vi "UDPPrototype.vi"() -> ()   [LabVIEW 2013, in "TEC tests.lvlib"]
uses:
  <vilib>/NI/Tag Bus/table/data table.ctl
  <vilib>/NI/Tag Bus/tag/Data Type.ctl
  <vilib>/NI/Tag Bus/tag/tag descriptor.lvclass
  <vilib>/NI/Tag Bus/dictionary/data dictionary.lvclass/data dictionary.ctl
  TEC tests.lvlib
  <vilib>/NI/Tag Bus/dictionary/data dictionary.lvclass
  <vilib>/NI/Tag Bus/table/data table.lvlib
panel:
  out "x = y?":bool
  out "error out":errorcluster
  in  "error in":errorcluster
  in  "Stop 2":bool
  out "Received Data":dbl(graph)
  in  "Stop":bool
  out "Current Data Value":dbl
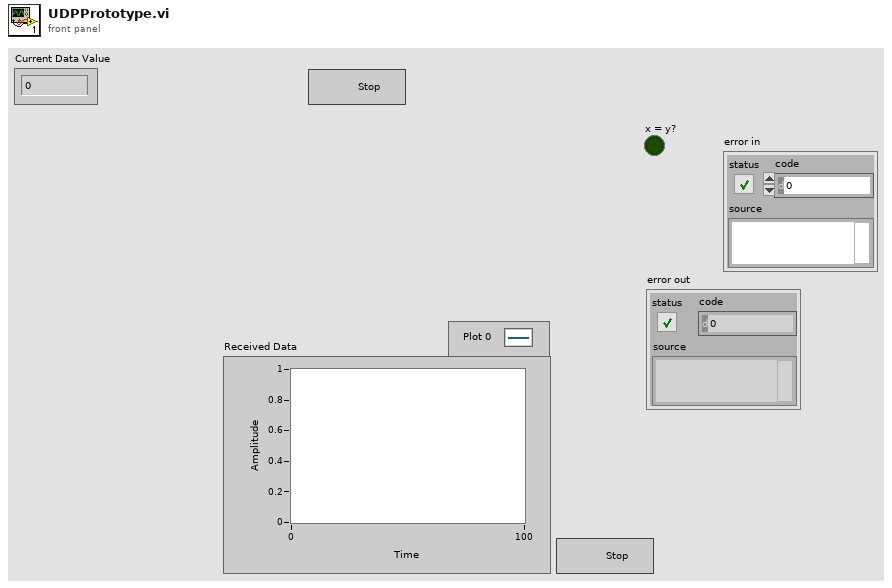
[diagram p1: front panel]
types:
  T1 = typedef "tag bus.lvlib/data table.lvlib/data table.ctl" = cluster{"Double":dbl[], "Single":sgl[], "I64":i64[], "I32":i32[], "I16":i16[], "I8":i8[], "U64":u64[], "U32":u32[], "U16":u16[], "U8":u8[], "Boolean":bool[], "String":string[], "Array of Double":cluster{"DBL Array":dbl[]}[], "Array of Single":cluster{"SGL Array":sgl[]}[], "Array of I64":cluster{"I64 Array":i64[]}[], "Array of I32":cluster{"I32 Array":i32[]}[], "Array of I16":cluster{"I16 Array":i16[]}[], "Array of I8":cluster{"I8 Array":i8[]}[], "Array of U64":cluster{"U64 Array":u64[]}[], "Array of U32":cluster{"U32 Array":u32[]}[], "Array of U16":cluster{"U16 Array":u16[]}[], "Array of U8":cluster{"U8 Array":u8[]}[], "Array of Boolean":cluster{"Boolean Array":bool[]}[], "Array of String":cluster{"String Array":string[]}[]}
  T2 = typedef "tag bus.lvlib/tag descriptor.lvclass/Data Type.ctl" = enum16{"Double", "Single", "I64", "I32", "I16", "I8", "U64", "U32", "U16", "U8", "Boolean", "String", "Array of Double", "Array of Single", "Array of I64", "Array of I32", "Array of I16", "Array of I8", "Array of U64", "Array of U32", "Array of U16", "Array of U8", "Array of Boolean", "Array of String"}
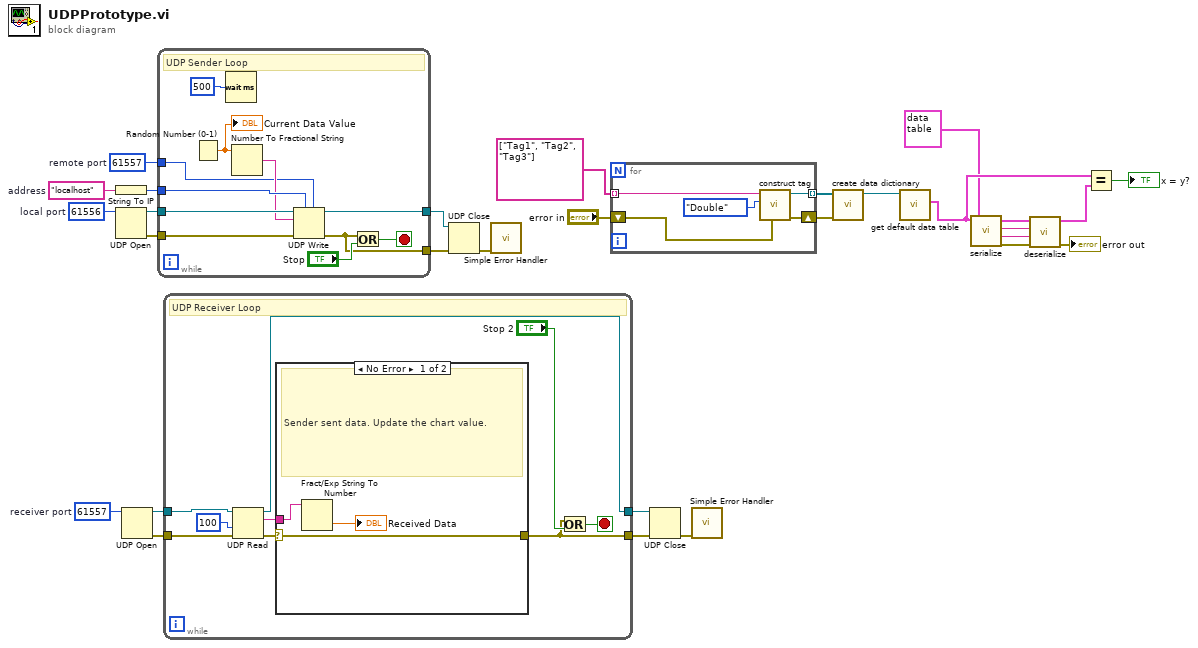
[diagram p0: block diagram]
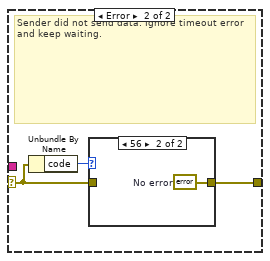
[diagram p2: hidden frame]
diagram:
  w14 = u16 61557  # receiver port
  w20 = u16 61557  # remote port
  w21 = u16 61556  # local port
  w26 = "localhost"  # address
  n1 = String To IP(1:w26) -> (0:w24:u32)
  n2 = UDP Open(11:w21) -> (port=w23:refnum<k16>, 0:w22:errorcluster)  [unwired: 4 in, 1 out]
  n3 = UDP Open(11:w14) -> (port=w15:refnum<k16>, 0:w16:errorcluster)  [unwired: 4 in, 1 out]
  n4 = while {
    tunnel: [w34] -> w27
    tunnel: w23 -> [w39]
    tunnel: w22 -> [w38]
    tunnel: [w35] -> w28
    tunnel: w24 -> [w33]
    tunnel: w20 -> [w30]
    stop <- w37 stop-if-true
    # "UDP Sender Loop"
    n5 = Random Number (0-1)() -> (number: 0 to 1=w29:dbl)
    "Current Data Value" <- w29
    n6 = Wait (ms)(milliseconds to wait=u32 500) -> ()  [unwired: 1 out]
    n7 = Number To Fractional String(number=w29) -> (F-format string=w31:string)  [unwired: 3 in]
    n8 = UDP Write(address=w33, port or service name=w30, connection ID=w39, data in=w31, 8:w38) -> (error out=w34:errorcluster, 3:w35:refnum<k16>)  [unwired: 1 in]
    n9 = Or(x=w34, y="Stop") -> (x .or. y?=w37:bool)
  }
  n10 = while {
    tunnel: w15 -> [w48]
    tunnel: [w40] -> w19
    tunnel: w16 -> [w45]
    tunnel: [w41] -> w17
    stop <- w46 stop-if-true
    # "UDP Receiver Loop"
    n11 = UDP Read(connection ID=w48, timeout ms (25000)=100, 8:w45) -> (data out=w43:string, error out=w42:errorcluster, 3:w40:refnum<k16>)  [unwired: 3 out]
    n12 = case shown="No Error" w42 {
      selector: w42 -> [w49 w53]
      tunnel: w43 -> [w51 _]
      tunnel: [w49 w52] -> w41
      frame No Error {
        # "Sender sent data. Update the chart value."
        n13 = Fract/Exp String To Number(string=w51) -> (number=→"Received Data":dbl)  [unwired: 3 in, 1 out]
      }
      frame Error {
        # "Sender did not send data. Ignore timeout error and keep waiting."
        n14 = Unbundle By Name(w53) -> ("code"=w54:i32)
        n15 = case shown="56" w54 {
          tunnel: w53 -> [w55 _]
          tunnel: [w55 w56] -> w52
          frame Default {
          }
          frame 56 {
            w56 = errorcluster {"status"=FALSE, "code"=0, "source"=""}  # No error
          }
        }
      }
    }
    n16 = Or(x=w41, y="Stop 2") -> (x .or. y?=w46:bool)
  }
  n17 = UDP Close(connection ID=w28, 8:w27) -> (error out=w25:errorcluster)  [unwired: 1 out]
  n18 = call <vilib>:"Simple Error Handler.vi"("error in (no error)"=w25) -> ()  [unwired: 4 in, 5 out]
  n19 = for {
    tunnel: [w61] -> w12 mode=indexing
    tunnel: string[] ["Tag1", "Tag2", "Tag3"] ("array") -> [w57] mode=indexing
    shift-right: [w58] -> w10
    shift-left: "error in" -> [w59]
    n20 = call <vilib>:"construct tag.vi"("error in"=w59, "data type"=Data_Type."Double", "name"=w57) -> ("error out"=w58:errorcluster, "system tag out"=w61:refnum<class "tag descriptor.lvclass">)  [unwired: 7 in]
  }
  n21 = UDP Close(connection ID=w19, 8:w17) -> (error out=w18:errorcluster)  [unwired: 1 out]
  n22 = call <vilib>:"Simple Error Handler.vi"("error in (no error)"=w18) -> ()  [unwired: 1 in, 8 out]
  n23 = call <vilib>:"create data dictionary.vi"("error in"=w10, "system tags"=w12) -> ("data dictionary"=w13:refnum<class "data dictionary.lvclass">)  [unwired: 8 in, 1 out]
  n24 = call <vilib>:"get default data table.vi"("data dictionary in"=w13) -> ("default data table"=w3:T1)  [unwired: 9 in, 1 out]
  n25 = call <vilib>:"serialize.vi"("data table in"=w3) -> ("error out"=w8:errorcluster, "data"=w6:string, "version"=w7:string)  [unwired: 7 in, 1 out]
  n26 = call <vilib>:"deserialize.vi"("error in"=w8, "data"=w6, "version"=w7, "data table in"=T1 {"Double"=[], "Single"=[], "I64"=[], "I32"=[], "I16"=[], "I8"=[], "U64"=[], "U32"=[], "U16"=[], "U8"=[], "Boolean"=[], "String"=[], "Array of Double"=[], "Array of Single"=[], "Array of I64"=[], "Array of I32"=[], "Array of I16"=[], "Array of I8"=[], "Array of U64"=[], "Array of U32"=[], "Array of U16"=[], "Array of U8"=[], "Array of Boolean"=[], "Array of String"=[]}) -> ("error out"=→"error out":errorcluster, "data table out"=w4:T1)  [unwired: 6 in]
  n27 = Equal?(x=w3, y=w4) -> (x = y?=→"x = y?":bool)
